vi "Stop Core.vi"(10 "final error code":i32, 11 "Storage in":refnum<class "Storage.lvclass">) -> (3 "Storage out":refnum<class "Storage.lvclass">)   [LabVIEW 2015, in "AMS UI.lvlib" / "Storage.lvclass"]
doc: "(<B>Filename</B>: Actor Framework.lvlib:Actor.lvclass:Stop Core.vi)\n\nDefines what the actor does before it stops. Use the <B>final error code</B> input to determine whether the actor shut down in response to an error.\n\nBy default, this method does nothing. A descendant class may override it to define behavior, such as shutting down any processes the actor initiated in its override of the Actor Core method."
uses:
  Storage.lvclass
  Storage.lvclass/Storage.ctl
  AMS Gas Actor/AMS Gas Actor.lvclass
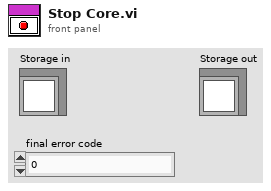
[diagram p1: front panel]
types:
  T1 = cluster{"Storage Line Control":refnum<k21>, "Storage Line Status":refnum<k21>}
  T2 = typedef "Sample Container.ctl" = cluster{"Sample In":refnum<k21>, "Sample Name":refnum<k21>, "Ti Cathode":refnum<k21>, "SampleQ":refnum<queue>}
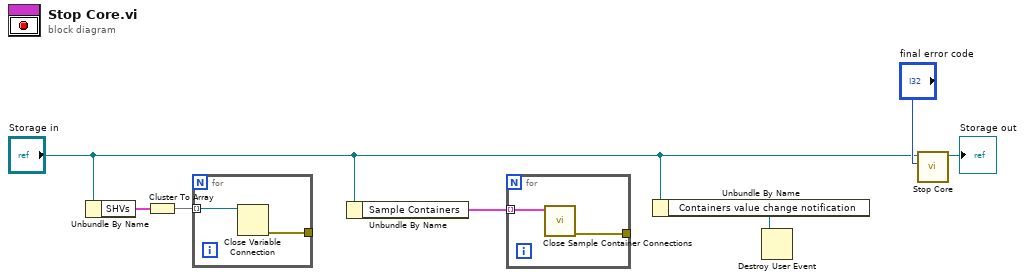
[diagram p0: block diagram]
diagram:
  n1 = Unbundle By Name("Storage in") -> ("SHVs"=w5:T1)
  n2 = Cluster To Array(cluster=w5) -> (array=w4:refnum<k21>[])
  n3 = for {
    tunnel: w4 -> [w9] mode=indexing
    tunnel: [w8] -> _
    n4 = Close Variable Connection(11:w9) -> (0:w8:errorcluster)  [unwired: 1 in]
  }
  n5 = Unbundle By Name("Storage in") -> ("Sample Containers"=w3:T2[])
  n6 = for {
    tunnel: w3 -> [w11] mode=indexing
    tunnel: [w10] -> _
    n7 = call "Close Sample Container Connections.vi"("Container in"=w11) -> ("error out"=w10:errorcluster)  [unwired: 9 in, 1 out]
  }
  n8 = Unbundle By Name("Storage in") -> ("Containers value change notification"=w1:refnum<user-event>)
  n9 = Destroy User Event(user event=w1) -> ()  [unwired: 1 in, 1 out]
  n10 = call-parent "Stop Core.vi"("final error code"="final error code", "AMS Gas Actor in"="Storage in") -> ("AMS Gas Actor out"=→"Storage out":refnum<class "Storage.lvclass">)  [unwired: 9 in]
